vi "SeqMgr.Data 2D Load from File.vi"(8 "error in (no error)":errorcluster, 11 "Args":string[](array[string])) -> (0 "error out":errorcluster, 1 "Max Indices":string[][](array[string]), 2 "Data":string[][](array[string]), 3 "Name":string)   [LabVIEW 2024, in "EQMF.lvlib" / "SeqMgr.lvlib"]
uses:
  SeqMgr.lvlib
  <vilib>/Utility/error.llb/Trim Whitespace One-Sided.vi
panel:
  # "Data2DLoadFromFile(VarName, MaxRow,MaxCol,Path,[Delimiter,ExcludeHeaderRowCnt])"
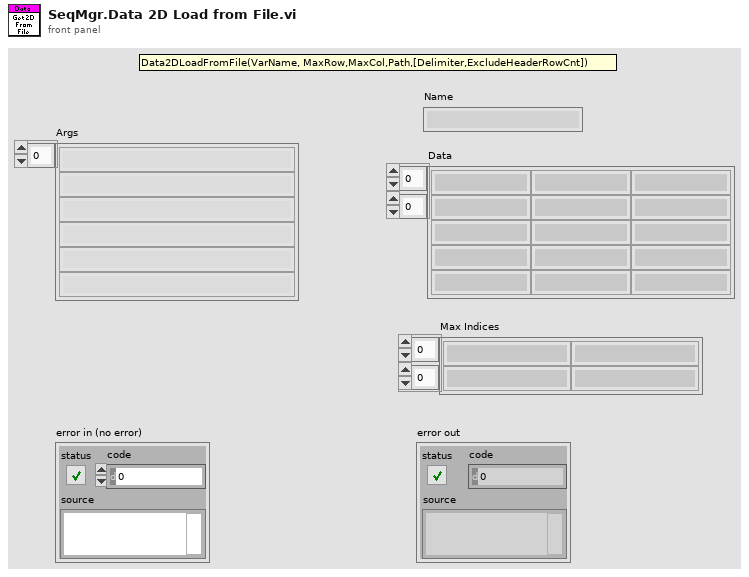
[diagram p1: front panel]
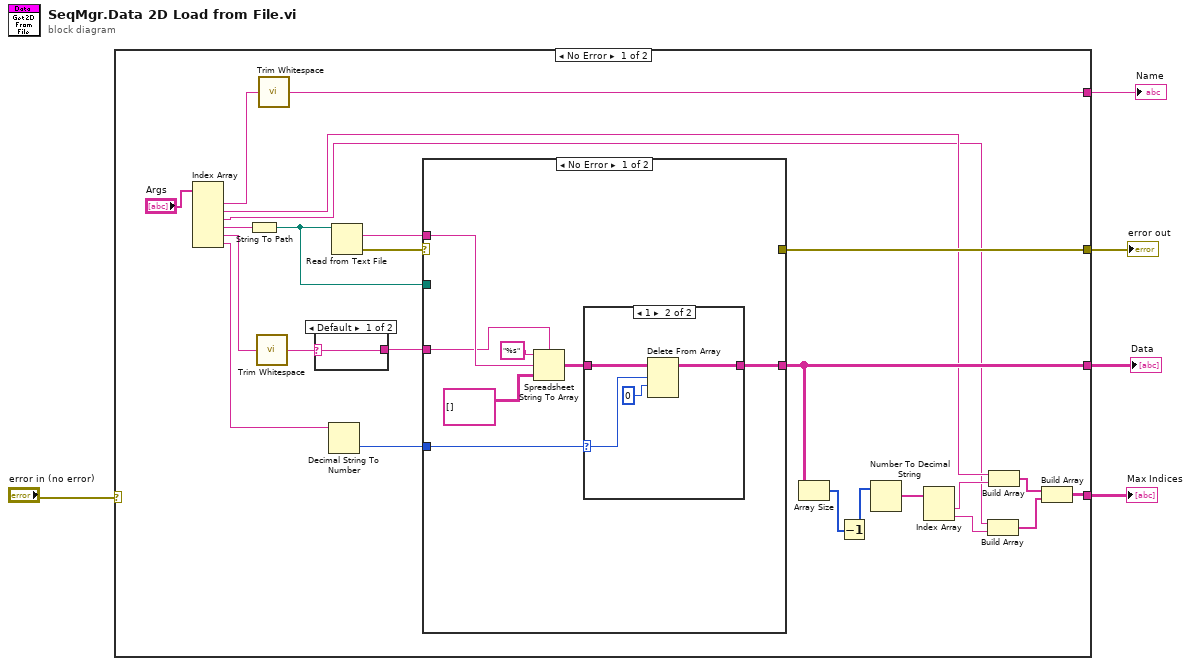
[diagram p0: block diagram]
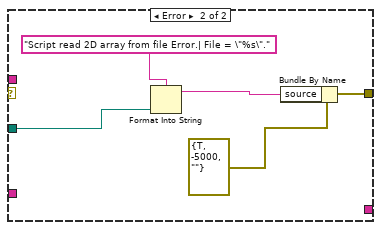
[diagram p3: hidden frame]
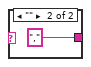
[diagram p4: hidden frame]
diagram:
  n1 = case shown="No Error" "error in (no error)" {
    selector: "error in (no error)" -> [_ w49]
    tunnel: [w22 _] -> w5
    tunnel: [w17 _] -> w4
    tunnel: [w19 w49] -> w3
    tunnel: [w14 _] -> w1
    frame No Error {
      n2 = Index Array(array="Args") -> (element #1=w16:string, element #2=w11:string, element #3=w9:string, element #4=w29:string, element #5=w27:string, element #6=w24:string)  [unwired: 6 in]
      n3 = String To Path(string=w29) -> (path=w18:path)
      n4 = call <vilib>:"Trim Whitespace.vi"("string"=w27) -> ("trimmed string"=w26:string)  [unwired: 1 in]
      n5 = call <vilib>:"Trim Whitespace.vi"("string"=w16) -> ("trimmed string"=w22:string)  [unwired: 1 in]
      n6 = case shown="Default" w26 {
        selector: w26 -> [w47 _]
        tunnel: [w47 ","] -> w25
        frame Default {
        }
        frame "" {
        }
      }
      n7 = Decimal String To Number(string=w24) -> (number=w21:i32)  [unwired: 2 in, 1 out]
      n8 = Read from Text File(file (use dialog)=w18) -> (text=w28:string, error out=w20:errorcluster)  [unwired: 3 in, 2 out]
      n9 = case shown="No Error" w20 {
        tunnel: w28 -> [w36 _]
        tunnel: w25 -> [w34 _]
        tunnel: w21 -> [w31 _]
        tunnel: [w30 _] -> w17
        tunnel: [_ w42] -> w19
        tunnel: w18 -> [_ w45]
        frame No Error {
          n10 = Spreadsheet String To Array(delimiter (Tab)=w34, format string="%s", spreadsheet string=w36, array type (2D Dbl)=string[][] [] ("Data")) -> (array=w32:string[][])
          n11 = case shown="1" w31 {
            selector: w31 -> [_ w40]
            tunnel: w32 -> [w37 w41]
            tunnel: [w37 w39] -> w30
            frame 0, Default {
            }
            frame 1 {
              n12 = Delete From Array(array=w41, length=w40, index (row)=0) -> (array with subset deleted=w39:string[][])  [unwired: 1 in, 1 out]
            }
          }
        }
        frame Error {
          n13 = Format Into String(format string="Script read 2D array from file Error.| File = \"%s\".", w45) -> (resulting string=w43:string)  [unwired: 2 in, 1 out]
          n14 = Bundle By Name(cluster=errorcluster {"status"=TRUE, "code"=-5000, "source"=""} ("error constant"), "source"=w43) -> (w42:errorcluster)
        }
      }
      n15 = Array Size(array=w17) -> (size(s)=w7:i32[])
      n16 = Decrement(x=w7) -> (x-1=w6:i32[])
      n17 = Number To Decimal String(number=w6) -> (decimal integer string=w15:string[])  [unwired: 1 in]
      n18 = Index Array(array=w15) -> (element #1=w13:string, element #2=w12:string)  [unwired: 2 in]
      n19 = Build Array(w9, w12) -> (w8:string[])
      n20 = Build Array(w11, w13) -> (w10:string[])
      n21 = Build Array(w10, w8) -> (w14:string[][])
    }
    frame Error {
    }
  }
  "Data" <- w4
  "error out" <- w3
  "Name" <- w5
  "Max Indices" <- w1
